vi "Bind Update Command Parameters.vi"(8 "Error In (no error)":errorcluster, 10 "Record":variant, 11 "SQL Statement In":refnum<class "SQL Statement.lvclass">) -> (0 "Error Out":errorcluster, 3 "SQL Statement Out":refnum<class "SQL Statement.lvclass">)   [LabVIEW 2023, in "SQLite DB Operator.lvclass"]
uses:
  SQLite DB Operator.lvclass
  <vilib>/drjdpowell/SQLite Library/SQL Statement/SQL Statement.lvclass
  DB Records/Expenses Tracker Balance/Public/Ctrls/Balance.ctl
  <vilib>/drjdpowell/SQLite Library/SQL Statement/SQL Statement.lvclass/SQL Statement.ctl
  DB Records/Expenses Tracker Category/Public/Ctrls/Category.ctl
  DB Records/Expenses Tracker Cycle/Public/Ctrls/Cycle.ctl
  DB Records/Expenses Tracker Saving Goal/Public/Ctrls/Saving Goal.ctl
  DB Records/Expenses Tracker Saving/Public/Ctrls/Saving.ctl
  DB Records/Expenses Tracker Subcategory/Public/Ctrls/Subcategory.ctl
  DB Records/Expenses Tracker Transaction/Public/Ctrls/Transaction.ctl
  <vilib>/drjdpowell/SQLite Library/SQL Statement/Bind Null.vi
  <vilib>/drjdpowell/SQLite Library/SQL Statement/Bind Timestamp (Real).vi
  <vilib>/drjdpowell/SQLite Library/SQL Statement/Bind Real.vi
  <vilib>/drjdpowell/SQLite Library/SQL Statement/Bind Integer.vi
  <vilib>/drjdpowell/SQLite Library/SQL Statement/Bind Text.vi
  <vilib>/drjdpowell/SQLite Library/SQL Statement/Error Message.vi
  DB Records/Expenses Tracker Category/Expenses Tracker Category.lvclass
  <vilib>/Utility/Data Type/NI_Data Type.lvlib
  DB Records/Expenses Tracker Transaction/Expenses Tracker Transaction.lvclass
  DB Records/Expenses Tracker Subcategory/Expenses Tracker Subcategory.lvclass
  DB Records/Expenses Tracker Balance/Expenses Tracker Balance.lvclass
  DB Records/Expenses Tracker Cycle/Expenses Tracker Cycle.lvclass
  DB Records/Expenses Tracker Saving Goal/Expenses Tracker Saving Goal.lvclass
  DB Records/Expenses Tracker Saving/Expenses Tracker Saving.lvclass
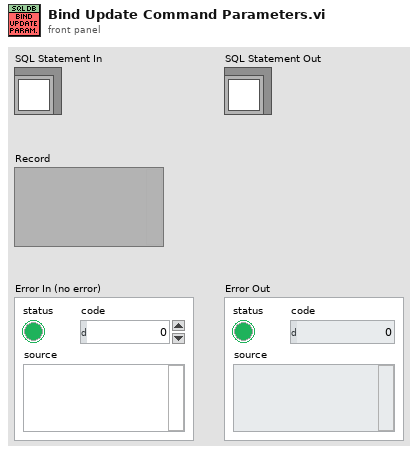
[diagram p1: front panel]
types:
  T1 = typedef "Expenses Tracker Balance.lvclass/Balance.ctl" = cluster{"ID":u8, "Value":dbl, "Last_update":timestamp}
  T2 = typedef "Expenses Tracker Category.lvclass/Category.ctl" = cluster{"ID":u32, "Name":string}
  T3 = typedef "Expenses Tracker Cycle.lvclass/Cycle.ctl" = cluster{"ID":u32, "Name":string, "Day_of_occurence":u8, "Description":string}
  T4 = typedef "Expenses Tracker Saving Goal.lvclass/Saving Goal.ctl" = cluster{"ID":u32, "Name":string, "Current_value":dbl, "Target_value":dbl, "Date_of_entry":timestamp, "Due_date":timestamp, "Last_update":timestamp, "Description":string}
  T5 = typedef "Expenses Tracker Saving.lvclass/Saving.ctl" = cluster{"ID":u32, "Saving_goal":u32, "Value":dbl, "Date_of_entry":timestamp, "Description":string}
  T6 = typedef "Expenses Tracker Subcategory.lvclass/Subcategory.ctl" = cluster{"ID":u32, "Name":string, "Category":u32}
  T7 = typedef "Expenses Tracker Transaction.lvclass/Transaction.ctl" = cluster{"ID":u32, "Name":string, "Is_income":bool, "Value":dbl, "Amount":dbl, "Total":dbl, "Date_of_entry":timestamp, "Date_of_occurence":timestamp, "Last_update":timestamp, "Category":u32, "Subcategory":u32, "Cycle":u32, "Description":string}
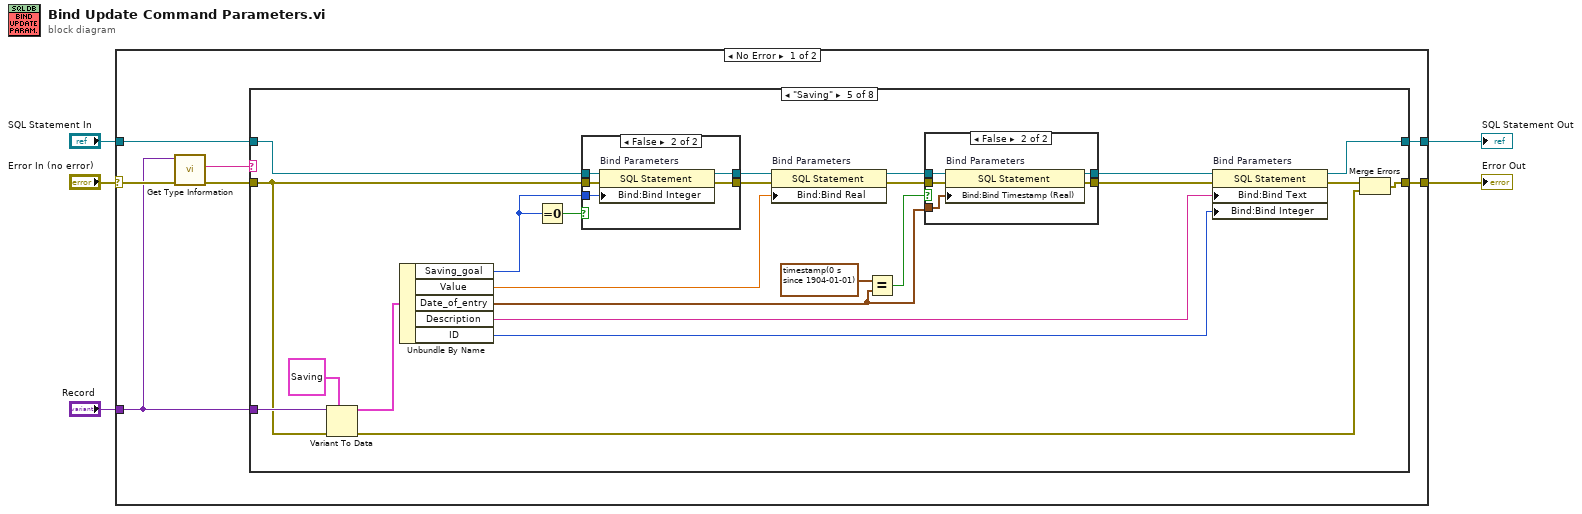
[diagram p0: block diagram]
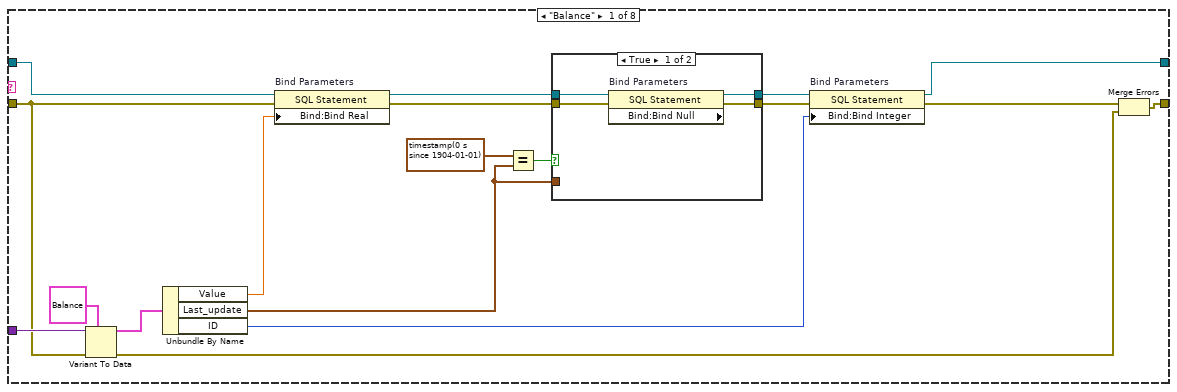
[diagram p2: hidden frame]
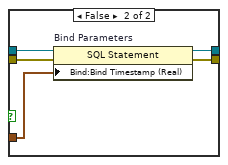
[diagram p3: hidden frame]
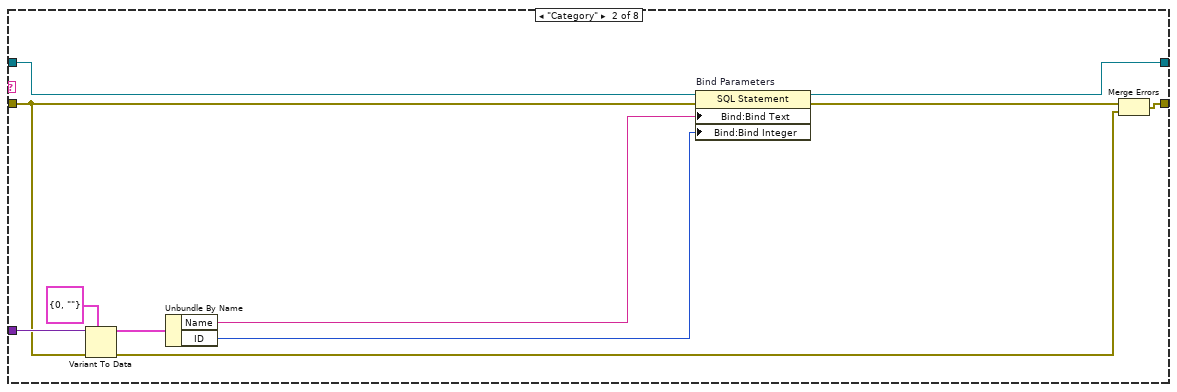
[diagram p4: hidden frame]
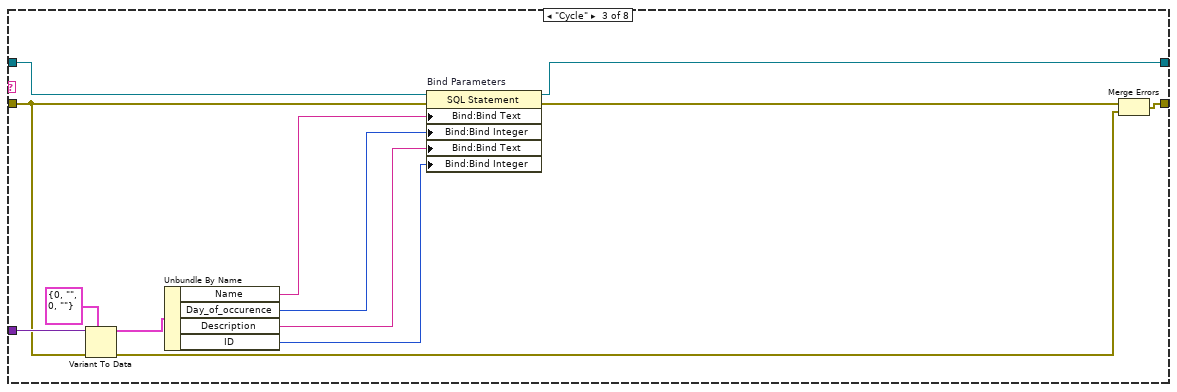
[diagram p5: hidden frame]
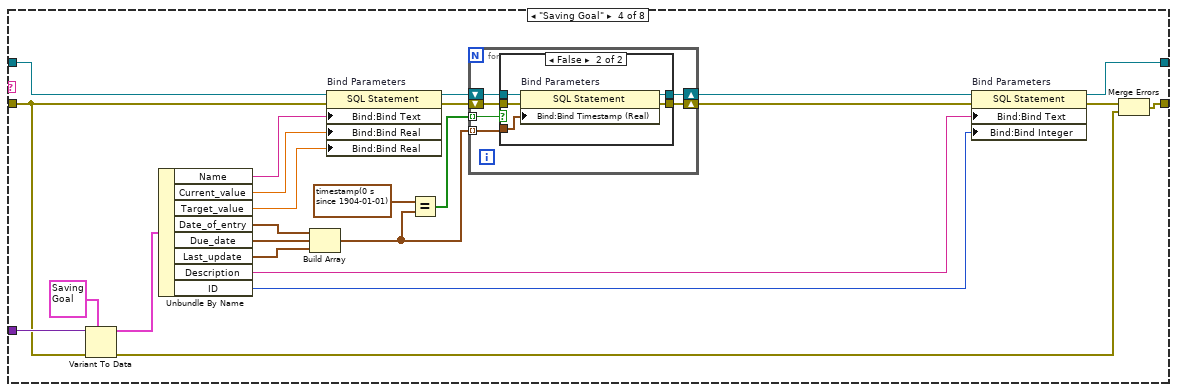
[diagram p6: hidden frame]
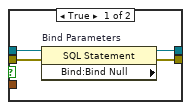
[diagram p7: hidden frame]
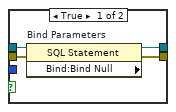
[diagram p8: hidden frame]
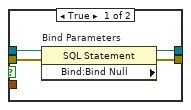
[diagram p9: hidden frame]
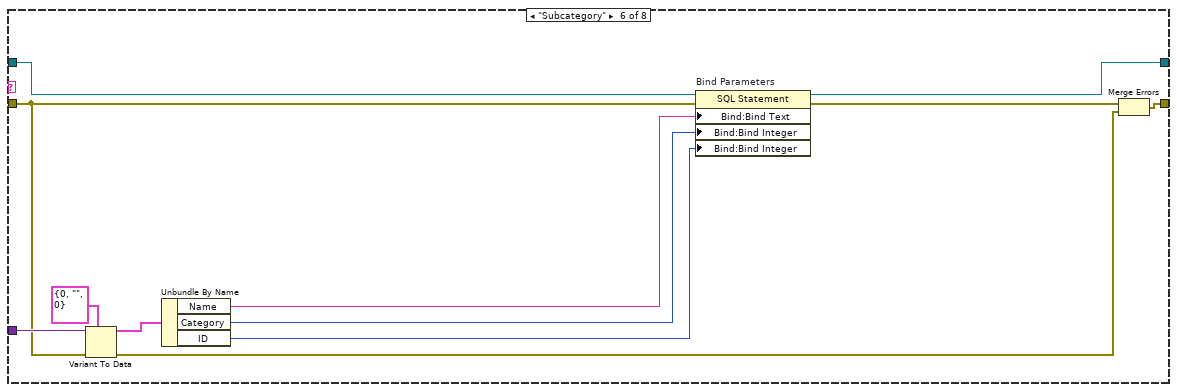
[diagram p10: hidden frame]
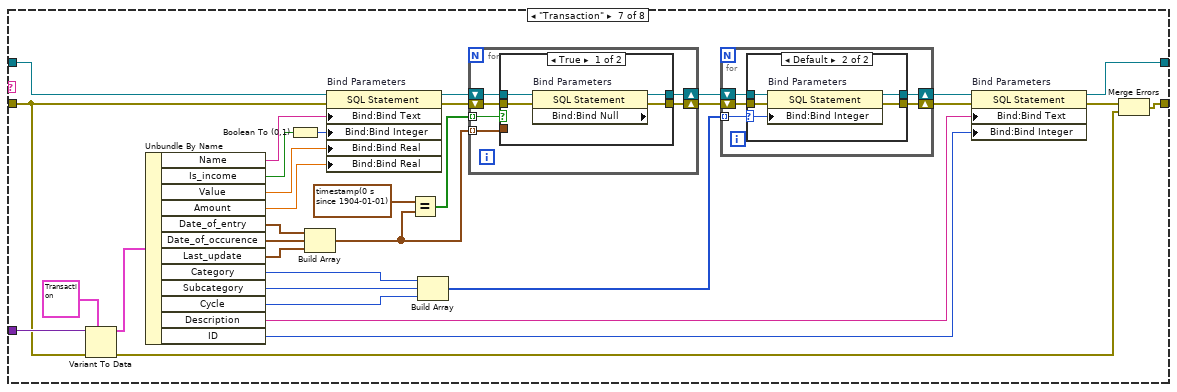
[diagram p11: hidden frame]
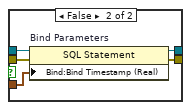
[diagram p12: hidden frame]
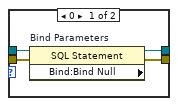
[diagram p13: hidden frame]
diagram:
  n1 = case shown="No Error" "Error In (no error)" {
    selector: "Error In (no error)" -> [w9 w219]
    tunnel: "SQL Statement In" -> [w12 w220]
    tunnel: [w11 w219] -> w4
    tunnel: [w10 w220] -> w3
    tunnel: "Record" -> [w8 _]
    frame No Error {
      n2 = call <vilib>:"Get Type Information.vi"("error in (no error)"=w9, "variant"=w8) -> ("error out"=w6:errorcluster, "name"=w7:string)  [unwired: 5 in, 3 out]
      n3 = case shown="\"Saving\"" w7 {
        tunnel: w8 -> [w30 w50 w63 w87 w125 w155 w187 _]
        tunnel: [w16 w49 w54 w80 w119 w154 w174 w218] -> w10
        tunnel: [w27 w44 w59 w83 w122 w149 w183 w217] -> w11
        tunnel: w12 -> [w24 w41 w56 w78 w117 w146 w167 w218]
        tunnel: w6 -> [w25 w42 w57 w79 w118 w147 w168 w217]
        frame "Balance" {
          n4 = Variant To Data(error in=w25, type=T1 {"ID"=0, "Value"=0.0, "Last_update"=timestamp(0 s since 1904-01-01)} ("Balance"), Variant=w30) -> (data=w29:T1, error out=w26:errorcluster)
          n5 = Unbundle By Name(w29) -> ("Value"=w18:dbl, "Last_update"=w19:timestamp, "ID"=w13:u8)
          n6 = property on="Bind Parameters" class="SQL Statement"(reference=w24, error in=w25, "Bind:Bind Real"=w18) -> (reference out=w22:refnum<class "SQL Statement.lvclass">, error out=w23:errorcluster)
          n7 = Equal?(x=timestamp(0 s since 1904-01-01), y=w19) -> (x = y?=w21:bool)
          n8 = case shown="True" w21 {
            tunnel: w23 -> [w34 w39]
            tunnel: w22 -> [w33 w38]
            tunnel: [w32 w37] -> w17
            tunnel: [w31 w36] -> w15
            tunnel: w19 -> [_ w35]
            frame True {
              n9 = property on="Bind Parameters" class="SQL Statement" props=["Bind:Bind Null"](reference=w33, error in=w34) -> (reference out=w32:refnum<class "SQL Statement.lvclass">, error out=w31:errorcluster)  [unwired: 1 out]
            }
            frame False {
              n10 = property on="Bind Parameters" class="SQL Statement"(reference=w38, error in=w39, "Bind:Bind Timestamp (Real)"=w35) -> (reference out=w37:refnum<class "SQL Statement.lvclass">, error out=w36:errorcluster)
            }
          }
          n11 = property on="Bind Parameters" class="SQL Statement"(reference=w17, error in=w15, "Bind:Bind Integer"=w13) -> (reference out=w16:refnum<class "SQL Statement.lvclass">, error out=w14:errorcluster)
          n12 = Merge Errors(w14, w26) -> (w27:errorcluster)
        }
        frame "Category" {
          n13 = Variant To Data(error in=w42, type=T2 {"ID"=0, "Name"=""} ("Category"), Variant=w50) -> (data=w47:T2, error out=w43:errorcluster)
          n14 = Unbundle By Name(w47) -> ("Name"=w45:string, "ID"=w40:u32)
          n15 = property on="Bind Parameters" class="SQL Statement"(reference=w41, error in=w42, "Bind:Bind Text"=w45, "Bind:Bind Integer"=w40) -> (reference out=w49:refnum<class "SQL Statement.lvclass">, error out=w48:errorcluster)
          n16 = Merge Errors(w48, w43) -> (w44:errorcluster)
        }
        frame "Cycle" {
          n17 = Variant To Data(error in=w57, type=T3 {"ID"=0, "Name"="", "Day_of_occurence"=0, "Description"=""} ("Cycle"), Variant=w63) -> (data=w62:T3, error out=w58:errorcluster)
          n18 = Unbundle By Name(w62) -> ("Name"=w60:string, "Day_of_occurence"=w53:u8, "Description"=w52:string, "ID"=w51:u32)
          n19 = property on="Bind Parameters" class="SQL Statement"(reference=w56, error in=w57, "Bind:Bind Text"=w60, "Bind:Bind Integer"=w53, "Bind:Bind Text"=w52, "Bind:Bind Integer"=w51) -> (reference out=w54:refnum<class "SQL Statement.lvclass">, error out=w55:errorcluster)
          n20 = Merge Errors(w55, w58) -> (w59:errorcluster)
        }
        frame "Saving Goal" {
          n21 = Variant To Data(error in=w79, type=T4 {"ID"=0, "Name"="", "Current_value"=0.0, "Target_value"=0.0, "Date_of_entry"=timestamp(0 s since 1904-01-01), "Due_date"=timestamp(0 s since 1904-01-01), "Last_update"=timestamp(0 s since 1904-01-01), "Description"=""} ("Saving Goal"), Variant=w87) -> (data=w86:T4, error out=w82:errorcluster)
          n22 = Unbundle By Name(w86) -> ("Name"=w84:string, "Current_value"=w70:dbl, "Target_value"=w69:dbl, "Date_of_entry"=w68:timestamp, "Due_date"=w67:timestamp, "Last_update"=w66:timestamp, "Description"=w65:string, "ID"=w64:u32)
          n23 = Build Array(w68, w67, w66) -> (w71:timestamp[])
          n24 = property on="Bind Parameters" class="SQL Statement"(reference=w78, error in=w79, "Bind:Bind Text"=w84, "Bind:Bind Real"=w70, "Bind:Bind Real"=w69) -> (reference out=w75:refnum<class "SQL Statement.lvclass">, error out=w74:errorcluster)
          n25 = Equal?(x=timestamp(0 s since 1904-01-01), y=w71) -> (x = y?=w72:bool[])
          n26 = for {
            shift-right: [w90] -> w77
            shift-left: w74 -> [w93]
            shift-right: [w91] -> w76
            shift-left: w75 -> [w92]
            tunnel: w72 -> [w89] mode=indexing
            tunnel: w71 -> [w88] mode=indexing
            n27 = case shown="False" w89 {
              tunnel: w93 -> [w97 w102]
              tunnel: w92 -> [w96 w101]
              tunnel: [w95 w100] -> w91
              tunnel: [w94 w99] -> w90
              tunnel: w88 -> [_ w98]
              frame True {
                n28 = property on="Bind Parameters" class="SQL Statement" props=["Bind:Bind Null"](reference=w96, error in=w97) -> (reference out=w95:refnum<class "SQL Statement.lvclass">, error out=w94:errorcluster)  [unwired: 1 out]
              }
              frame False {
                n29 = property on="Bind Parameters" class="SQL Statement"(reference=w101, error in=w102, "Bind:Bind Timestamp (Real)"=w98) -> (reference out=w100:refnum<class "SQL Statement.lvclass">, error out=w99:errorcluster)
              }
            }
          }
          n30 = property on="Bind Parameters" class="SQL Statement"(reference=w76, error in=w77, "Bind:Bind Text"=w65, "Bind:Bind Integer"=w64) -> (reference out=w80:refnum<class "SQL Statement.lvclass">, error out=w81:errorcluster)
          n31 = Merge Errors(w81, w82) -> (w83:errorcluster)
        }
        frame "Saving" {
          n32 = Variant To Data(error in=w118, type=T5 {"ID"=0, "Saving_goal"=0, "Value"=0.0, "Date_of_entry"=timestamp(0 s since 1904-01-01), "Description"=""} ("Saving"), Variant=w125) -> (data=w124:T5, error out=w121:errorcluster)
          n33 = Unbundle By Name(w124) -> ("Saving_goal"=w104:u32, "Value"=w106:dbl, "Date_of_entry"=w111:timestamp, "Description"=w112:string, "ID"=w103:u32)
          n34 = Equal To 0?(x=w104) -> (x = 0?=w105:bool)
          n35 = case shown="False" w105 {
            tunnel: w104 -> [_ w134]
            tunnel: w118 -> [w129 w133]
            tunnel: w117 -> [w128 w132]
            tunnel: [w127 w131] -> w110
            tunnel: [w126 w130] -> w109
            frame True {
              n36 = property on="Bind Parameters" class="SQL Statement" props=["Bind:Bind Null"](reference=w128, error in=w129) -> (reference out=w127:refnum<class "SQL Statement.lvclass">, error out=w126:errorcluster)  [unwired: 1 out]
            }
            frame False {
              n37 = property on="Bind Parameters" class="SQL Statement"(reference=w132, error in=w133, "Bind:Bind Integer"=w134) -> (reference out=w131:refnum<class "SQL Statement.lvclass">, error out=w130:errorcluster)
            }
          }
          n38 = property on="Bind Parameters" class="SQL Statement"(reference=w110, error in=w109, "Bind:Bind Real"=w106) -> (reference out=w107:refnum<class "SQL Statement.lvclass">, error out=w108:errorcluster)
          n39 = Equal?(x=timestamp(0 s since 1904-01-01), y=w111) -> (x = y?=w113:bool)
          n40 = case shown="False" w113 {
            tunnel: w108 -> [w138 w143]
            tunnel: w107 -> [w137 w142]
            tunnel: [w136 w141] -> w115
            tunnel: [w135 w140] -> w116
            tunnel: w111 -> [_ w139]
            frame True {
              n41 = property on="Bind Parameters" class="SQL Statement" props=["Bind:Bind Null"](reference=w137, error in=w138) -> (reference out=w136:refnum<class "SQL Statement.lvclass">, error out=w135:errorcluster)  [unwired: 1 out]
            }
            frame False {
              n42 = property on="Bind Parameters" class="SQL Statement"(reference=w142, error in=w143, "Bind:Bind Timestamp (Real)"=w139) -> (reference out=w141:refnum<class "SQL Statement.lvclass">, error out=w140:errorcluster)
            }
          }
          n43 = property on="Bind Parameters" class="SQL Statement"(reference=w115, error in=w116, "Bind:Bind Text"=w112, "Bind:Bind Integer"=w103) -> (reference out=w119:refnum<class "SQL Statement.lvclass">, error out=w120:errorcluster)
          n44 = Merge Errors(w120, w121) -> (w122:errorcluster)
        }
        frame "Subcategory" {
          n45 = Variant To Data(error in=w147, type=T6 {"ID"=0, "Name"="", "Category"=0} ("Subcategory"), Variant=w155) -> (data=w152:T6, error out=w148:errorcluster)
          n46 = Unbundle By Name(w152) -> ("Name"=w150:string, "Category"=w145:u32, "ID"=w144:u32)
          n47 = property on="Bind Parameters" class="SQL Statement"(reference=w146, error in=w147, "Bind:Bind Text"=w150, "Bind:Bind Integer"=w145, "Bind:Bind Integer"=w144) -> (reference out=w154:refnum<class "SQL Statement.lvclass">, error out=w153:errorcluster)
          n48 = Merge Errors(w153, w148) -> (w149:errorcluster)
        }
        frame "Transaction" {
          n49 = Variant To Data(error in=w168, type=T7 {"ID"=0, "Name"="", "Is_income"=FALSE, "Value"=0.0, "Amount"=0.0, "Total"=0.0, "Date_of_entry"=timestamp(0 s since 1904-01-01), "Date_of_occurence"=timestamp(0 s since 1904-01-01), "Last_update"=timestamp(0 s since 1904-01-01), "Category"=0, "Subcategory"=0, "Cycle"=0, "Description"=""} ("Transaction"), Variant=w187) -> (data=w186:T7, error out=w182:errorcluster)
          n50 = Unbundle By Name(w186) -> ("Name"=w184:string, "Is_income"=w179:bool, "Value"=w180:dbl, "Amount"=w181:dbl, "Date_of_entry"=w162:timestamp, "Date_of_occurence"=w161:timestamp, "Last_update"=w160:timestamp, "Category"=w172:u32, "Subcategory"=w171:u32, "Cycle"=w170:u32, "Description"=w173:string, "ID"=w156:u32)
          n51 = Boolean To (0,1)(Boolean=w179) -> (0, 1=w178:i16)
          n52 = Build Array(w162, w161, w160) -> (w157:timestamp[])
          n53 = property on="Bind Parameters" class="SQL Statement"(reference=w167, error in=w168, "Bind:Bind Text"=w184, "Bind:Bind Integer"=w178, "Bind:Bind Real"=w180, "Bind:Bind Real"=w181) -> (reference out=w164:refnum<class "SQL Statement.lvclass">, error out=w163:errorcluster)
          n54 = Equal?(x=timestamp(0 s since 1904-01-01), y=w157) -> (x = y?=w158:bool[])
          n55 = Build Array(w172, w171, w170) -> (w169:u32[])
          n56 = for {
            shift-right: [w190] -> w166
            shift-left: w163 -> [w193]
            shift-right: [w191] -> w165
            shift-left: w164 -> [w192]
            tunnel: w158 -> [w189] mode=indexing
            tunnel: w157 -> [w188] mode=indexing
            n57 = case shown="True" w189 {
              tunnel: w193 -> [w197 w202]
              tunnel: w192 -> [w196 w201]
              tunnel: [w195 w200] -> w191
              tunnel: [w194 w199] -> w190
              tunnel: w188 -> [_ w198]
              frame True {
                n58 = property on="Bind Parameters" class="SQL Statement" props=["Bind:Bind Null"](reference=w196, error in=w197) -> (reference out=w195:refnum<class "SQL Statement.lvclass">, error out=w194:errorcluster)  [unwired: 1 out]
              }
              frame False {
                n59 = property on="Bind Parameters" class="SQL Statement"(reference=w201, error in=w202, "Bind:Bind Timestamp (Real)"=w198) -> (reference out=w200:refnum<class "SQL Statement.lvclass">, error out=w199:errorcluster)
              }
            }
          }
          n60 = for {
            shift-right: [w204] -> w176
            shift-left: w166 -> [w207]
            shift-right: [w205] -> w177
            shift-left: w165 -> [w206]
            tunnel: w169 -> [w203] mode=indexing
            n61 = case shown="Default" w203 {
              selector: w203 -> [_ w212]
              tunnel: w207 -> [w211 w216]
              tunnel: w206 -> [w210 w215]
              tunnel: [w209 w214] -> w205
              tunnel: [w208 w213] -> w204
              frame 0 {
                n62 = property on="Bind Parameters" class="SQL Statement" props=["Bind:Bind Null"](reference=w210, error in=w211) -> (reference out=w209:refnum<class "SQL Statement.lvclass">, error out=w208:errorcluster)  [unwired: 1 out]
              }
              frame Default {
                n63 = property on="Bind Parameters" class="SQL Statement"(reference=w215, error in=w216, "Bind:Bind Integer"=w212) -> (reference out=w214:refnum<class "SQL Statement.lvclass">, error out=w213:errorcluster)
              }
            }
          }
          n64 = property on="Bind Parameters" class="SQL Statement"(reference=w177, error in=w176, "Bind:Bind Text"=w173, "Bind:Bind Integer"=w156) -> (reference out=w174:refnum<class "SQL Statement.lvclass">, error out=w175:errorcluster)
          n65 = Merge Errors(w175, w182) -> (w183:errorcluster)
        }
        frame Default {
        }
      }
    }
    frame Error {
    }
  }
  "Error Out" <- w4
  "SQL Statement Out" <- w3
